vi "Decode SSL Wrapper Package.vi"(5 "Version":string(combo)="Auto", 8 "error in (no error)":errorcluster, 9 "FIRASim?":bool=TRUE, 10 "Ignore left/rigth?":bool[](array[boolean]), 11 "unsigned byte array":u8[](array[numeric])) -> (0 "error out":errorcluster, 1 "Geometry Camera Calibration":T2, 2 "Field":T1, 3 "Detection Frame":T3 {"robots_blue"."height" format="%+4.3f"; "robots_blue"."pixel_y" format="%+4.3f"; "robots_blue"."pixel_x" format="%+4.3f"; "robots_blue"."orientation" format="%+4.3f"; "robots_blue"."y" format="%+4.3f"; "robots_blue"."confidence" format="%4.3f"; "robots_blue"."x" format="%+4.3f"; "robots_yellow"."height" format="%+4.3f"; "robots_yellow"."pixel_y" format="%+4.3f"; "robots_yellow"."pixel_x" format="%+4.3f"; "robots_yellow"."orientation" format="%+4.3f"; "robots_yellow"."y" format="%+4.3f"; "robots_yellow"."confidence" format="%4.3f"; "robots_yellow"."x" format="%+4.3f"}, 4 "Empty Field Size?":bool, 6 "Empty Information?":bool)   [LabVIEW 2020]
uses:
  Varint Decoder uint32.vi
  Robot_class/FieldFIRASim.ctl
  Controls/SSL Detection Robot.ctl
  Controls/SSL Detection Ball.ctl
  Controls/SSL Detection Frame.ctl
  Controls/SSL Geometry Camera Calibration.ctl
  <vilib>/Analysis/Matrix/Datatypes/RealMatrix.ctl
  <vilib>/Analysis/Matrix/NI_Matrix.lvlib
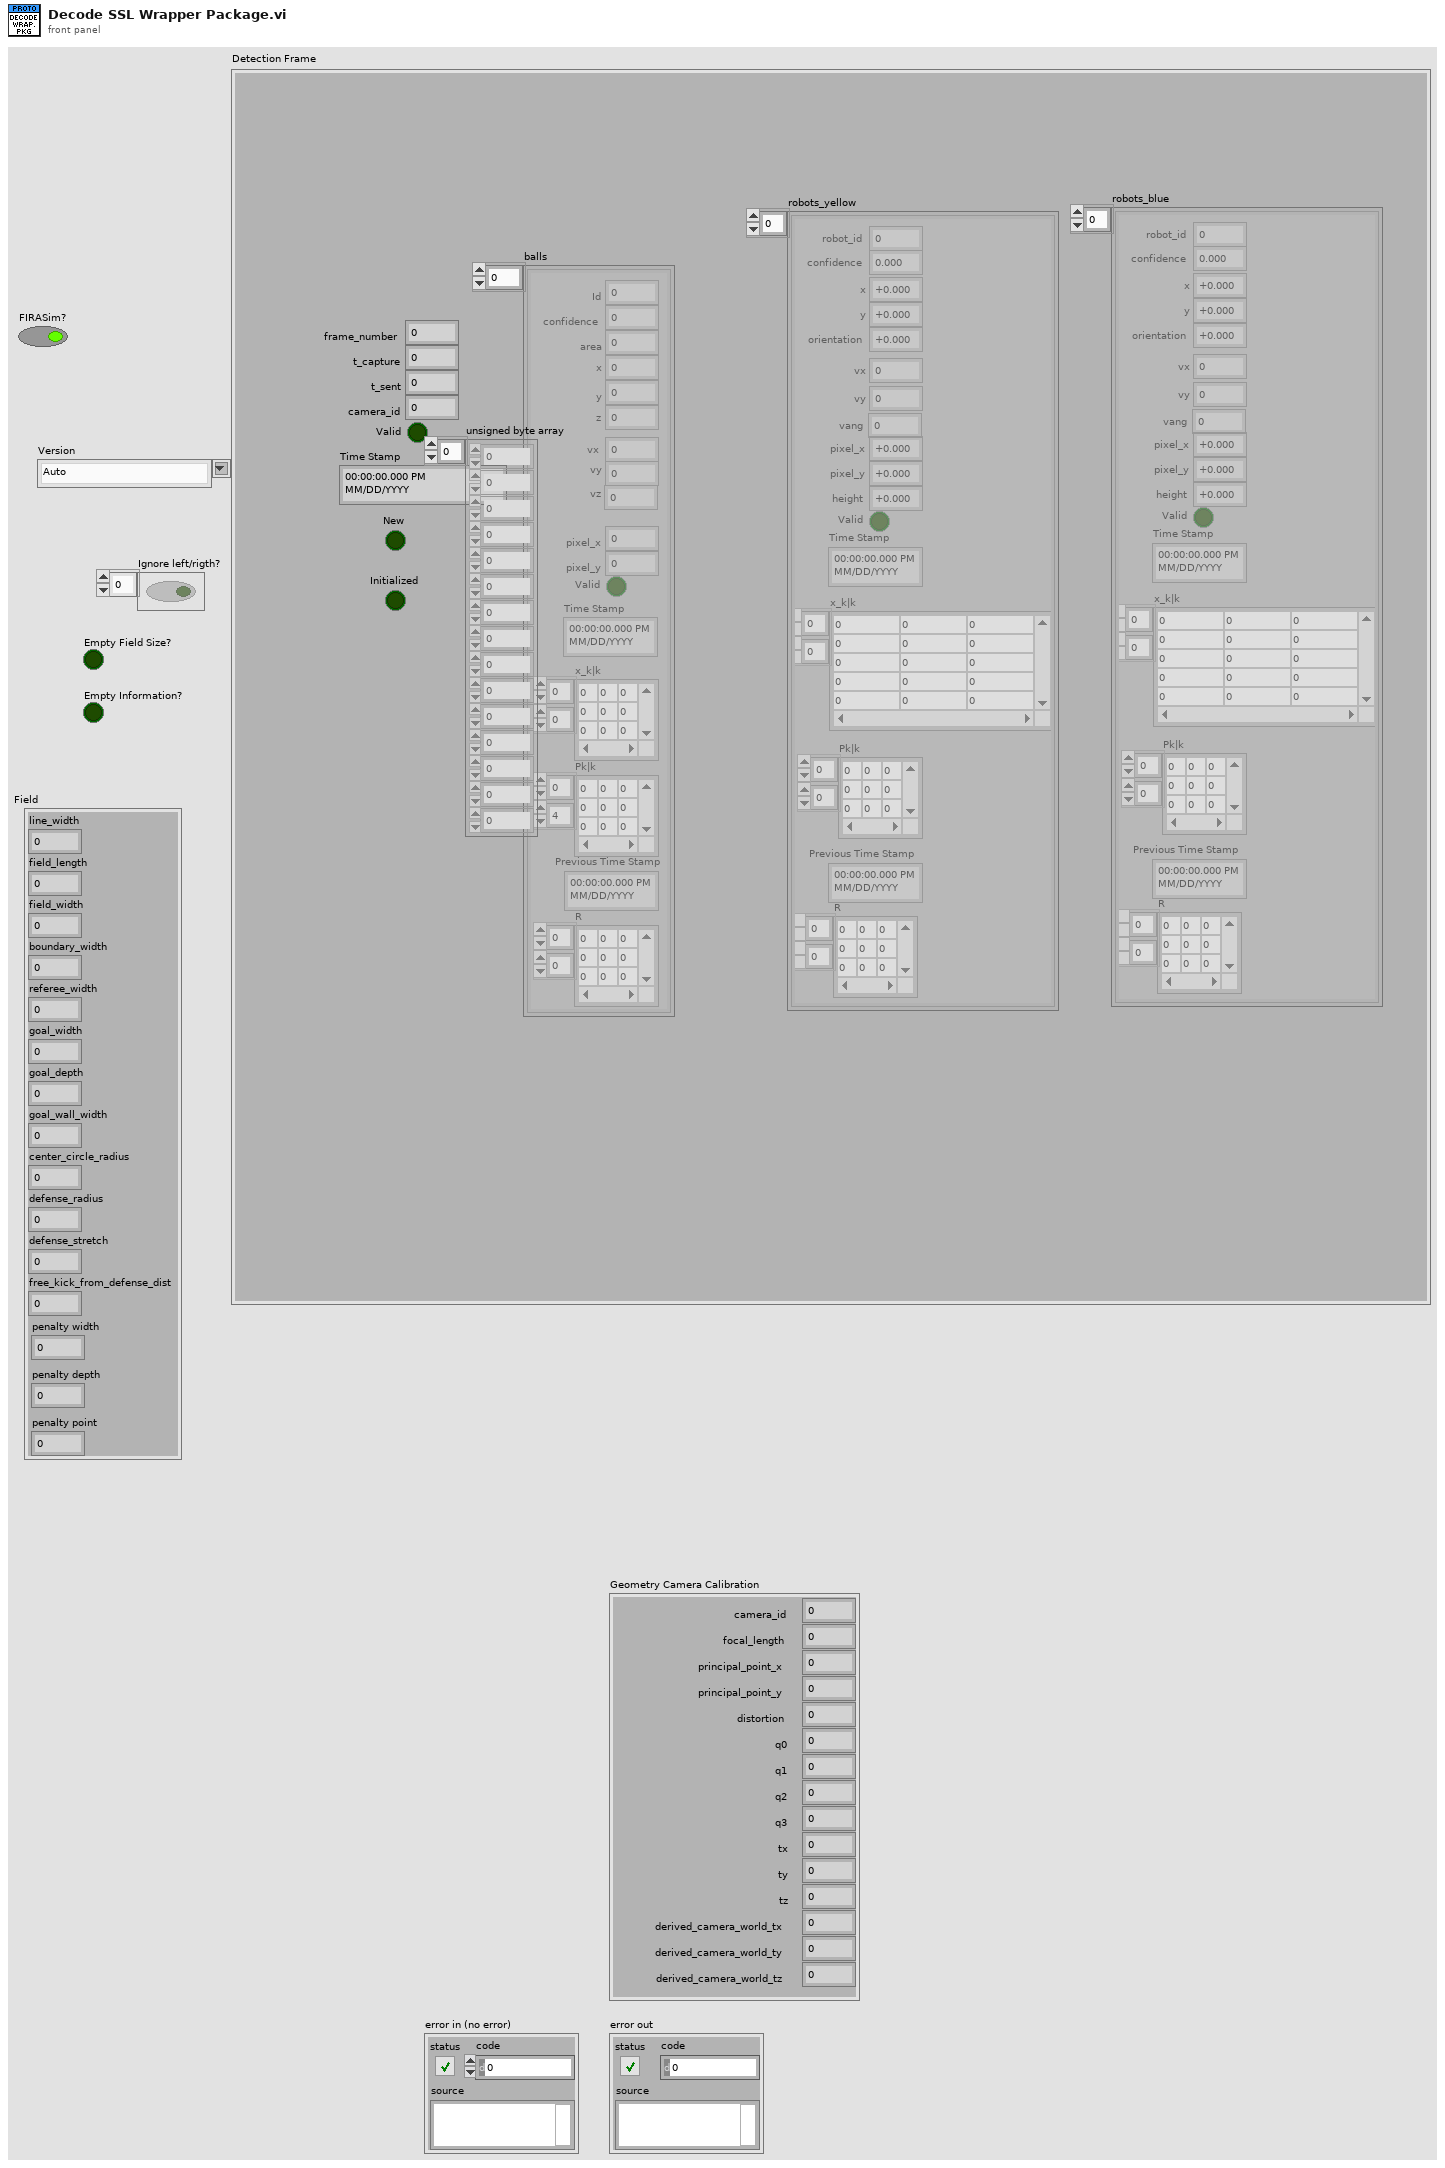
[diagram p1: front panel]
types:
  T1 = typedef "FieldFIRASim.ctl" = cluster{"line_width":u32, "field_length":u32, "field_width":u32, "boundary_width":u32, "referee_width":u32, "goal_width":u32, "goal_depth":u32, "goal_wall_width":u32, "center_circle_radius":u32, "defense_radius":u32, "defense_stretch":u32, "free_kick_from_defense_dist":u32, "penalty width":dbl, "penalty depth":dbl, "penalty point":dbl}
  T2 = typedef "SSL Geometry Camera Calibration.ctl" = cluster{"camera_id":u32, "focal_length":sgl, "principal_point_x":sgl, "principal_point_y":sgl, "distortion":sgl, "q0":sgl, "q1":sgl, "q2":sgl, "q3":sgl, "tx":sgl, "ty":sgl, "tz":sgl, "derived_camera_world_tx":sgl, "derived_camera_world_ty":sgl, "derived_camera_world_tz":sgl}
  T3 = typedef "SSL Detection Frame.ctl" = cluster{"frame_number":u32, "t_capture":dbl, "t_sent":dbl, "camera_id":u32, "robots_yellow":T4[], "robots_blue":T4[], "balls":T6[], "Valid":bool, "Time Stamp":timestamp, "New":bool, "Initialized":bool}
  T4 = typedef "SSL Detection Robot.ctl" = cluster{"x":sgl, "robot_id":u32, "confidence":sgl, "y":sgl, "orientation":sgl, "pixel_x":sgl, "pixel_y":sgl, "height":sgl, "Valid":bool, "Time Stamp":timestamp, "x_k|k":T5, "Pk|k":T5, "Previous Time Stamp":timestamp, "R":T5, "vx":dbl, "vy":dbl, "vang":dbl}
  T5 = typedef "NI_Matrix.lvlib/RealMatrix.ctl" = dbl[][]
  T6 = typedef "SSL Detection Ball.ctl" = cluster{"x":sgl, "area":u32, "confidence":sgl, "y":sgl, "z":sgl, "pixel_x":sgl, "pixel_y":sgl, "Valid":bool, "Time Stamp":timestamp, "x_k|k":T5, "Pk|k":T5, "Id":u32, "Previous Time Stamp":timestamp, "R":T5, " vx":sgl, "vy":dbl, "vz":dbl}
  T7 = cluster{"line_width":u32, "field_length":u32, "field_width":u32, "boundary_width":u32, "referee_width":u32, "goal_width":u32, "goal_depth":u32, "goal_wall_width":u32, "center_circle_radius":u32, "defense_radius":u32, "defense_stretch":u32, "free_kick_from_defense_dist":u32, "penalty_spot_from_field_line_dist":u32, "penalty_line_from_spot_dist":u32}
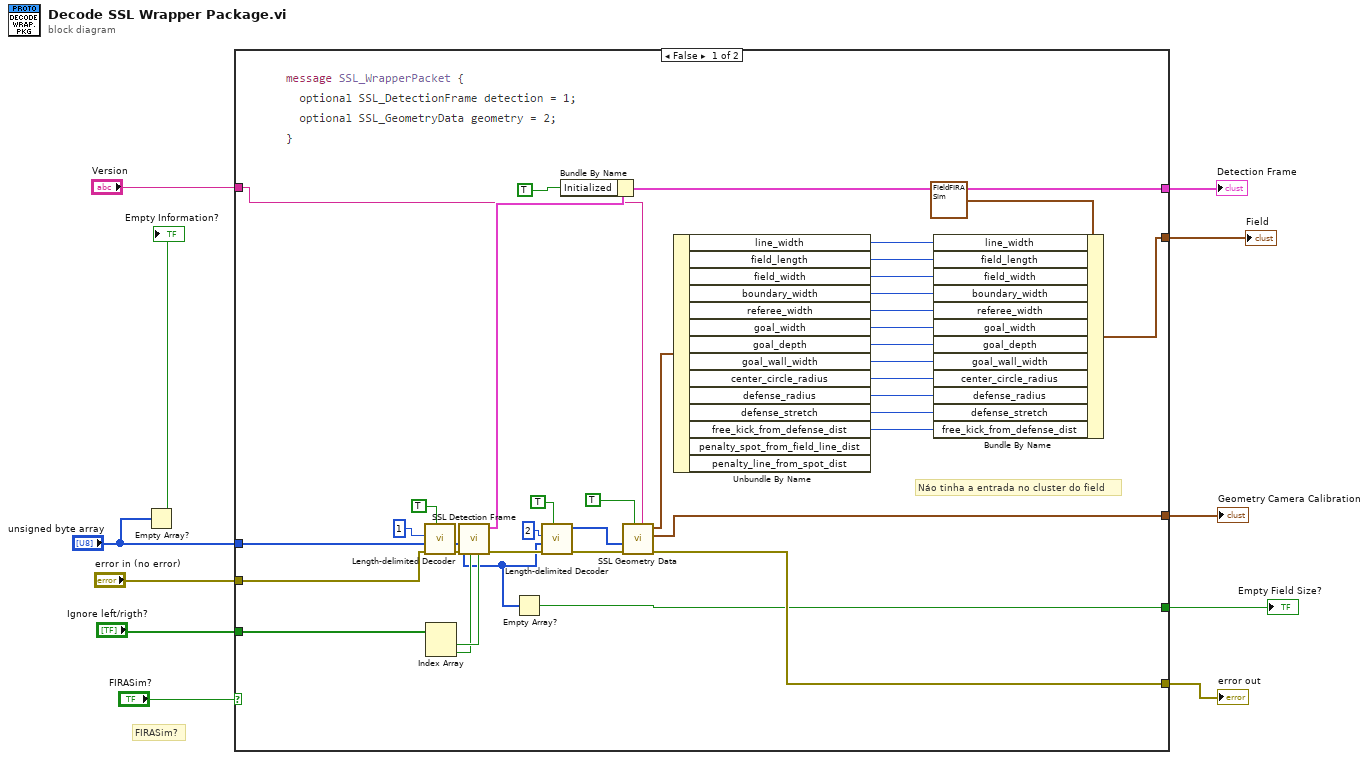
[diagram p0: block diagram]
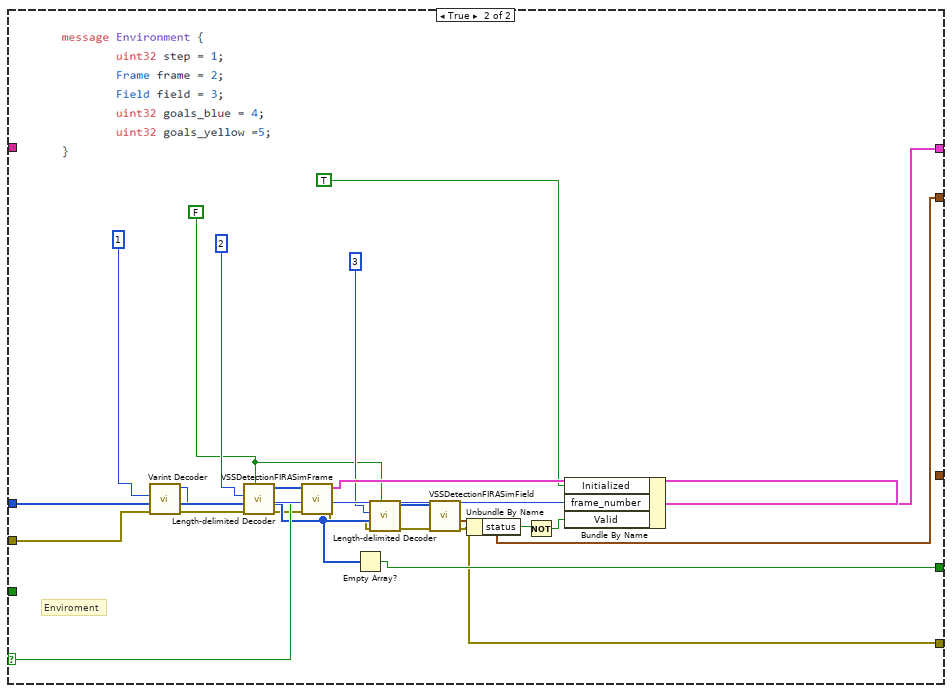
[diagram p2: hidden frame]
diagram:
  # "FIRASim?"
  n1 = Empty Array?(array="unsigned byte array") -> (empty?=→"Empty Information?":bool)
  n2 = case shown="False" "FIRASim?" {
    selector: "FIRASim?" -> [_ w65]
    tunnel: [w49 w55] -> w11
    tunnel: "Ignore left/rigth?" -> [w38 _]
    tunnel: [w25 w50] -> w1
    tunnel: [w35 _] -> w4
    tunnel: [w33 w61] -> w9
    tunnel: [w31 w66] -> w7
    tunnel: "unsigned byte array" -> [w29 w67]
    tunnel: "error in (no error)" -> [w28 w58]
    tunnel: "Version" -> [w27 _]
    frame False {
      # "Náo tinha a entrada no cluster do field"
      n3 = call "Length-delimited Decoder.vi"("Optional"=TRUE, "error in (no error)"=w28, "Array"=w29, "Key"=1) -> ("error out"=w41:errorcluster, "array w/ subset deleted"=w34:u8[], "Length-delimited"=w44:u8[])  [unwired: 4 in, 1 out]
      n4 = Index Array(array=w38) -> (element #1=w37:bool, element #2=w36:bool)  [unwired: 2 in]
      n5 = call "SSL Detection Frame.vi"("ignora esquerda?"=w37, "ignora direita?"=w36, "error in"=w41, "Array"=w44) -> ("error out"=w42:errorcluster, "Detection Frame"=w32:T3)  [unwired: 6 in]
      n6 = Empty Array?(array=w34) -> (empty?=w33:bool)
      n7 = call "Length-delimited Decoder.vi"("Optional"=TRUE, "error in (no error)"=w42, "Array"=w34, "Key"=2) -> ("error out"=w43:errorcluster, "Length-delimited"=w47:u8[])  [unwired: 4 in, 2 out]
      n8 = Bundle By Name(cluster=w32, "Initialized"=TRUE) -> (w31:T3)
      n9 = call "SSL Geometry Data.vi"("Version"=w27, "Optional"=TRUE, "error in"=w43, "Array"=w47) -> ("error out"=w49:errorcluster, "Geometry Camera Calibration"=w35:T2, "Field Size"=w26:T7)  [unwired: 5 in]
      n10 = Unbundle By Name(w26) -> ("line_width"=w23:u32, "field_length"=w22:u32, "field_width"=w21:u32, "boundary_width"=w20:u32, "referee_width"=w19:u32, "goal_width"=w18:u32, "goal_depth"=w17:u32, "goal_wall_width"=w16:u32, "center_circle_radius"=w15:u32, "defense_radius"=w14:u32, "defense_stretch"=w13:u32, "free_kick_from_defense_dist"=w12:u32)  [unwired: 2 out]
      n11 = Bundle By Name(cluster=T1 {"line_width"=0, "field_length"=0, "field_width"=0, "boundary_width"=0, "referee_width"=0, "goal_width"=0, "goal_depth"=0, "goal_wall_width"=0, "center_circle_radius"=0, "defense_radius"=0, "defense_stretch"=0, "free_kick_from_defense_dist"=0, "penalty width"=0.0, "penalty depth"=0.0, "penalty point"=0.0} ("Field 2"), "line_width"=w23, "field_length"=w22, "field_width"=w21, "boundary_width"=w20, "referee_width"=w19, "goal_width"=w18, "goal_depth"=w17, "goal_wall_width"=w16, "center_circle_radius"=w15, "defense_radius"=w14, "defense_stretch"=w13, "free_kick_from_defense_dist"=w12) -> (w25:T1)
    }
    frame True {
      w51 = FALSE ("Optional")
      # "Enviroment"
      n12 = call-poly "Varint Decoder.vi"("error in (no error)"=w58, "Array"=w67, "Key"=1) -> ("error out"=w60:errorcluster, "array w/ subset deleted"=w72:u8[], "Varint"=w68:u32)  [unwired: 5 in, 1 out]
      n13 = call "Length-delimited Decoder.vi"("Optional"=w51, "error in (no error)"=w60, "Array"=w72, "Key"=2) -> ("error out"=w59:errorcluster, "array w/ subset deleted"=w62:u8[], "Length-delimited"=w70:u8[])  [unwired: 4 in, 1 out]
      n14 = call "VSSDetectionFIRASimFrame.vi"("error in (no error)"=w59, "FIRASim?"=w65, "Frame"=w70) -> ("error out"=w57:errorcluster, "Detection Frame out"=w69:T3)  [unwired: 7 in]
      n15 = Empty Array?(array=w62) -> (empty?=w61:bool)
      n16 = call "Length-delimited Decoder.vi"("Optional"=w51, "error in (no error)"=w57, "Array"=w62, "Key"=3) -> ("error out"=w56:errorcluster, "Length-delimited"=w63:u8[])  [unwired: 4 in, 2 out]
      n17 = call "VSSDetectionFIRASimField.vi"("error in (no error)"=w56, "Field"=w63) -> ("error out"=w55:errorcluster, "Field"=w50:T1)  [unwired: 7 in, 1 out]
      n18 = Unbundle By Name(w55) -> ("status"=w54:bool)
      n19 = Not(x=w54) -> (.not. x?=w53:bool)
      n20 = Bundle By Name(cluster=w69, "Initialized"=TRUE, "frame_number"=w68, "Valid"=w53) -> (w66:T3)
    }
  }
  "Detection Frame" <- w7
  "error out" <- w11
  "Geometry Camera Calibration" <- w4
  "Empty Field Size?" <- w9
  "Field" <- w1
